vi "Disconnect.vi"(8 "error in (no error)":errorcluster, 11 "controller":refnum<k24>) -> (0 "error out":errorcluster)   [LabVIEW 2016]
uses:
  C:/Users/Aerotech/Documents/BNLStaveAssembly-blueprint/Bin/Aerotech.A3200.dll
  Bin/Aerotech.A3200.dll
  C:/Users/Aerotech/Documents/BNLStaveAssembly-blueprint/Bin/Aerotech.A3200.LabVIEW.dll
  Bin/Aerotech.A3200.LabVIEW.dll
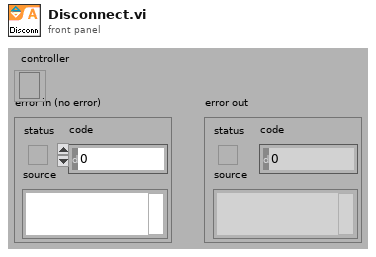
[diagram p1: front panel]
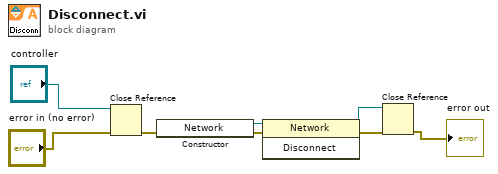
[diagram p0: block diagram]
diagram:
  n1 = Close Reference(reference="controller", error in (no error)="error in (no error)") -> (error out=w2:errorcluster)
  n2 = constructor class="Network"(error in=w2) -> (reference out=w3:refnum<k24>, error out=w7:errorcluster)  [unwired: 2 in, 1 out]
  n3 = invoke class="Network" method="Disconnect"(reference=w3, error in=w7) -> (reference out=w4:refnum<k24>, error out=w6:errorcluster)  [unwired: 1 in, 1 out]
  n4 = Close Reference(reference=w4, error in (no error)=w6) -> (error out=→"error out":errorcluster)
